vi "循环脉冲脚本.vi"(4 "4-wire":bool, 6 "脉冲":T1 {"测试参数"."反向极限电流(mA)" min=0.0 max=3000.0; "测试参数"."反向电压(V)" min=-40.0 max=40.0; "测试参数"."读取电压(V)" min=-40.0 max=40.0; "测试参数"."正向极限电流(mA)" min=0.0 max=3000.0; "测试参数"."正向电压(V)" min=-40.0 max=40.0}, 8 "错误输入（无错误）":errorcluster, 11 "循环次数":u32) -> (0 "错误输出":errorcluster, 1 "Script":string)   [LabVIEW 2020, in "功能选择.xctl"]
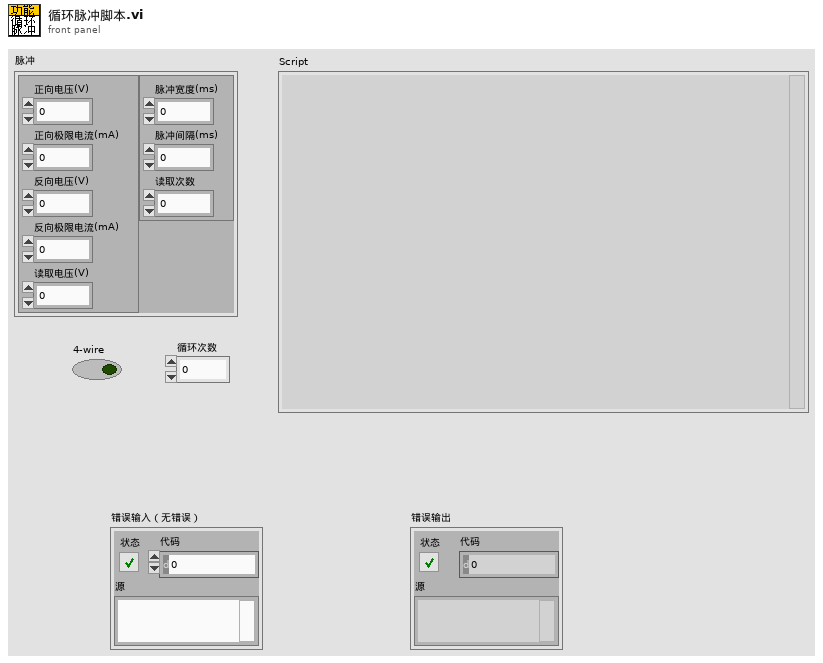
[diagram p1: front panel]
types:
  T1 = typedef "功能选择.xctl/脉冲参数.ctl" = cluster{"测试参数":cluster{"正向电压(V)":dbl, "正向极限电流(mA)":dbl, "反向电压(V)":dbl, "反向极限电流(mA)":dbl, "读取电压(V)":dbl}, "时序参数":cluster{"脉冲宽度(ms)":dbl, "脉冲间隔(ms)":dbl, "读取次数":u32}}
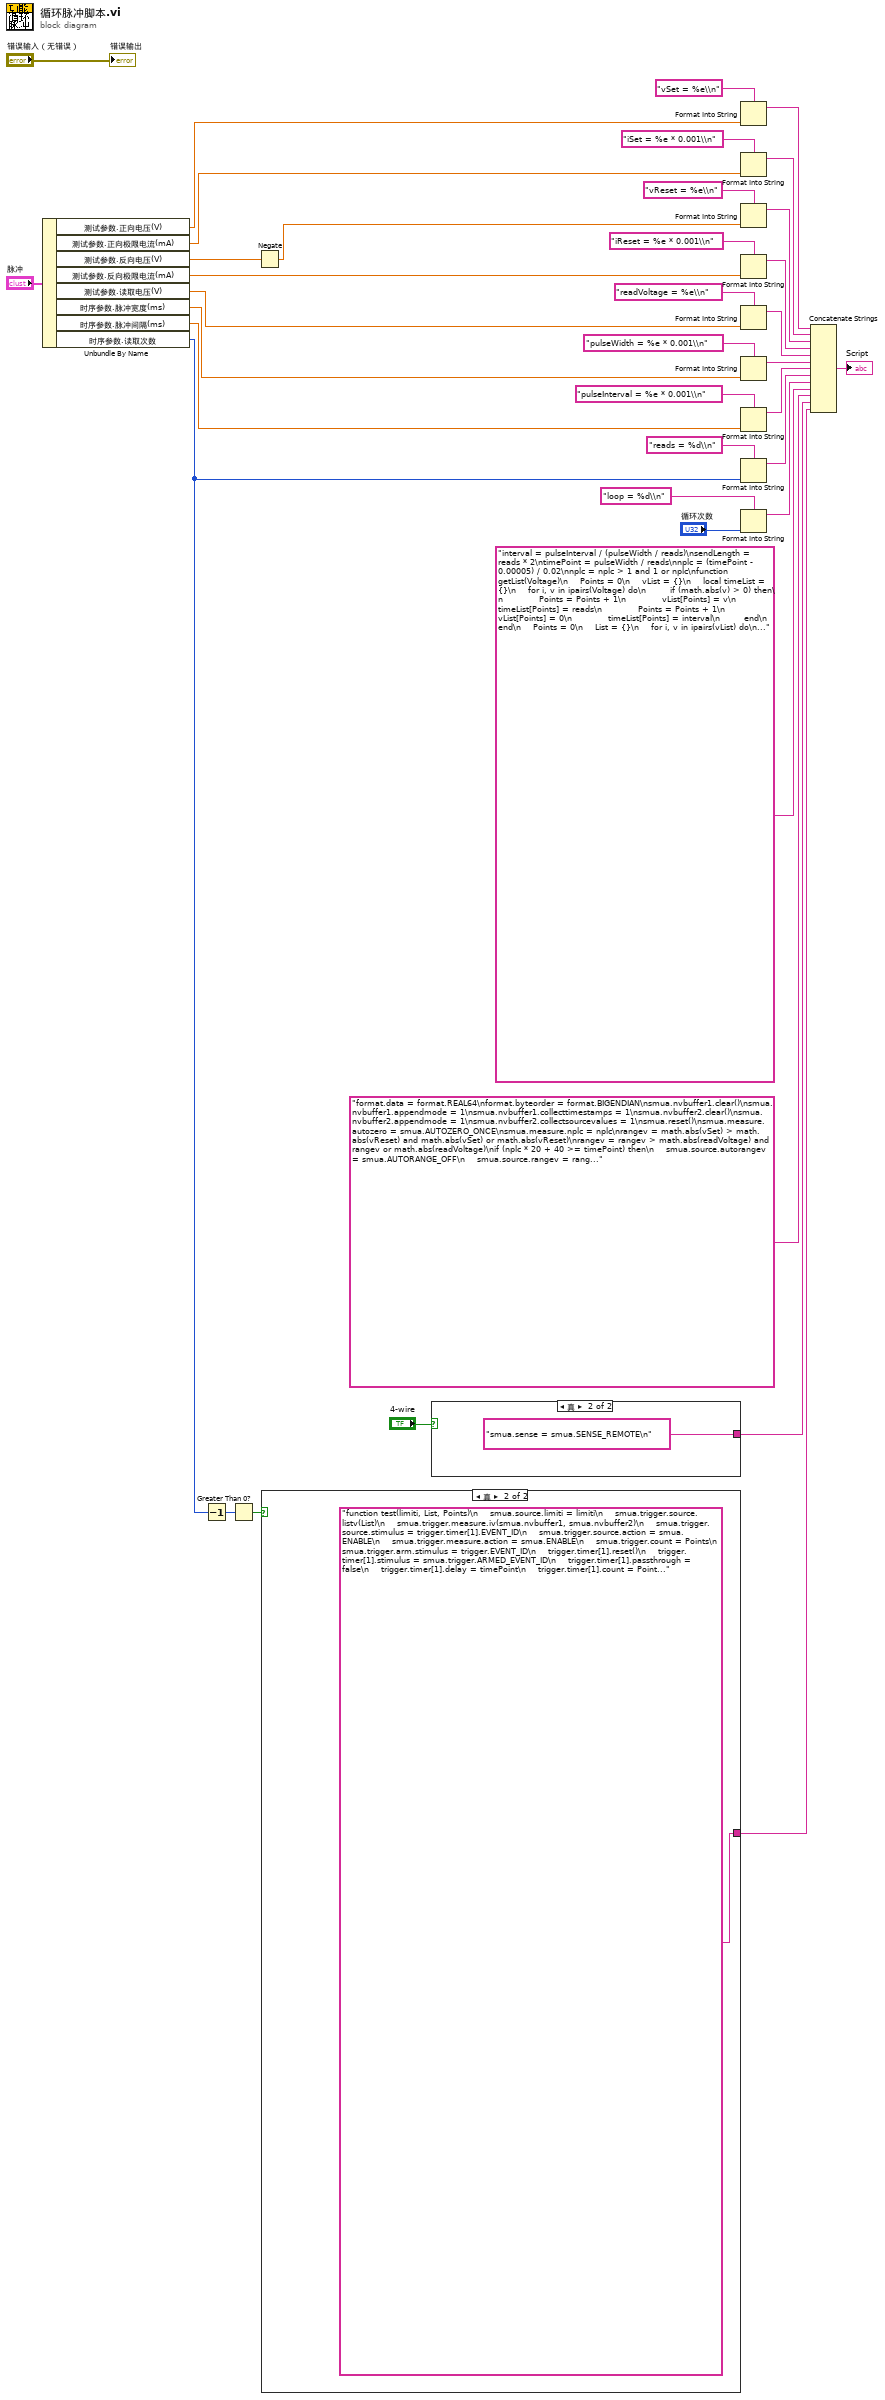
[diagram p0: block diagram]
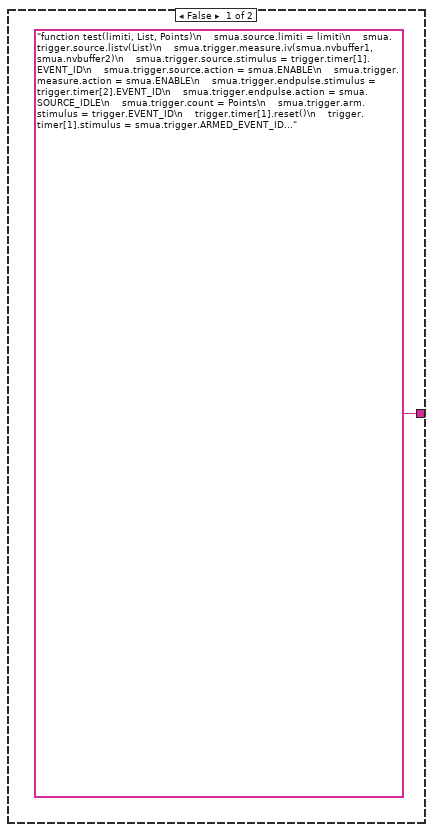
[diagram p2: hidden frame]
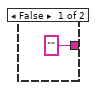
[diagram p3: hidden frame]
diagram:
  n1 = Unbundle By Name("脉冲") -> ("测试参数.正向电压(V)"=w24:dbl, "测试参数.正向极限电流(mA)"=w23:dbl, "测试参数.反向电压(V)"=w22:dbl, "测试参数.反向极限电流(mA)"=w21:dbl, "测试参数.读取电压(V)"=w30:dbl, "时序参数.脉冲宽度(ms)"=w29:dbl, "时序参数.脉冲间隔(ms)"=w2:dbl, "时序参数.读取次数"=w9:u32)
  n2 = Decrement(x=w9) -> (x-1=w10:u32)
  n3 = Greater Than 0?(x=w10) -> (x > 0?=w6:bool)
  n4 = Negate(x=w22) -> (-x=w8:dbl)
  n5 = case shown="真" w6 {
    tunnel: ["function test(limiti, List, Points)\n    smua.source.limiti = limiti\n    smua.trigger.source.listv(List)\n    smua.trigger.measure.iv(smua.nvbuffer1, smua.nvbuffer2)\n    smua.trigger.source.stimulus = trigger.timer[1].EVENT_ID\n    smua.trigger.source.action = smua.ENABLE\n    smua.trigger.measure.action = smua.ENABLE\n    smua.trigger.endpulse.stimulus = trigger.timer[2].EVENT_ID\n    smua.trigger.endpulse.action = smua.SOURCE_IDLE\n    smua.trigger.count = Points\n    smua.trigger.arm.stimulus = trigger.EVENT_ID\n    trigger.timer[1].reset()\n    trigger.timer[1].stimulus = smua.trigger.ARMED_EVENT_ID\n    trigger.timer[1].passthrough = false\n    trigger.timer[1].delay = timePoint\n    trigger.timer[1].count = Points\n    trigger.timer[2].reset()\n    trigger.timer[2].stimulus = trigger.timer[1].EVENT_ID\n    trigger.timer[2].passthrough = false\n    trigger.timer[2].delay = pulseWidth\n    trigger.timer[2].count = 1\n    smua.trigger.initiate()\n    smua.trigger.arm.set()\nend\nsmua.source.output = smua.OUTPUT_ON\nfor i = 1, loop do\n    if (setPoints > 0) then\n        test(iSet, setList, setPoints)\n        waitcomplete()\n    end\n    if (ResetPoints > 0) then\n        test(iReset, ResetList, ResetPoints)\n        waitcomplete()\n    end\nend\nsmua.source.output = smua.OUTPUT_OFF\nStart = 1\nStop = smua.nvbuffer1.n\nprint(\"{\" .. Stop .. \"}\")\nprintbuffer(Start, Stop, smua.nvbuffer1.timestamps)\nprintbuffer(Start, Stop, smua.nvbuffer2.sourcevalues)\nprintbuffer(Start, Stop, smua.nvbuffer1)\nprintbuffer(Start, Stop, smua.nvbuffer2)\nprint(\"{done}\")\nreset()" ("字符串") "function test(limiti, List, Points)\n    smua.source.limiti = limiti\n    smua.trigger.source.listv(List)\n    smua.trigger.measure.iv(smua.nvbuffer1, smua.nvbuffer2)\n    smua.trigger.source.stimulus = trigger.timer[1].EVENT_ID\n    smua.trigger.source.action = smua.ENABLE\n    smua.trigger.measure.action = smua.ENABLE\n    smua.trigger.count = Points\n    smua.trigger.arm.stimulus = trigger.EVENT_ID\n    trigger.timer[1].reset()\n    trigger.timer[1].stimulus = smua.trigger.ARMED_EVENT_ID\n    trigger.timer[1].passthrough = false\n    trigger.timer[1].delay = timePoint\n    trigger.timer[1].count = Points\n    smua.trigger.initiate()\n    smua.trigger.arm.set()\nend\nfunction sendData()\n    repeat\n        if (bit.test(status.operation.instrument.smua.condition, 4) == false) then\n            return\n        elseif (smua.nvbuffer1.n > Stop) then\n            print(\"{\" .. sendLength .. \"}\")\n            printbuffer(Start, Stop, smua.nvbuffer1.timestamps)\n            printbuffer(Start, Stop, smua.nvbuffer2.sourcevalues)\n            printbuffer(Start, Stop, smua.nvbuffer1)\n            printbuffer(Start, Stop, smua.nvbuffer2)\n            Start = Start + sendLength\n            Stop = Stop + sendLength\n        end\n        delay(timePoint)\n    until (false)\nend\nfunction sendLastData()\n    Stop = smua.nvbuffer1.n\n    print(\"{\" .. Stop - Start + 1 .. \"}\")\n    printbuffer(Start, Stop, smua.nvbuffer1.timestamps)\n    printbuffer(Start, Stop, smua.nvbuffer2.sourcevalues)\n    printbuffer(Start, Stop, smua.nvbuffer1)\n    printbuffer(Start, Stop, smua.nvbuffer2)\n    print(\"{done}\")\nend\nStart = 1\nStop = sendLength\nsmua.source.output = smua.OUTPUT_ON\ntest(iSet, startList, startPoints)\nsendData()\nfor i = 1, loop do\n    if (setPoints > 0) then\n        test(iSet, setList, setPoints)\n        sendData()\n    end\n    if (ResetPoints > 0) then\n        test(iReset, ResetList, ResetPoints)\n        sendData()\n    end\nend\nsmua.source.output = smua.OUTPUT_OFF\nsendLastData()\nreset()" ("字符串")] -> w13
    frame False {
    }
    frame True {
    }
  }
  n6 = case shown="真" "4-wire" {
    tunnel: ["" "smua.sense = smua.SENSE_REMOTE\n"] -> w36
    frame False {
    }
    frame True {
    }
  }
  n7 = Format Into String(format string="vSet = %e\\n" ("格式字符串"), w24) -> (resulting string=w20:string)  [unwired: 2 in, 1 out]
  n8 = Format Into String(format string="iSet = %e * 0.001\\n" ("格式字符串"), w23) -> (resulting string=w19:string)  [unwired: 2 in, 1 out]
  n9 = Format Into String(format string="vReset = %e\\n" ("格式字符串"), w8) -> (resulting string=w18:string)  [unwired: 2 in, 1 out]
  n10 = Format Into String(format string="iReset = %e * 0.001\\n" ("格式字符串"), w21) -> (resulting string=w17:string)  [unwired: 2 in, 1 out]
  n11 = Format Into String(format string="readVoltage = %e\\n" ("格式字符串"), w30) -> (resulting string=w16:string)  [unwired: 2 in, 1 out]
  n12 = Format Into String(format string="pulseWidth = %e * 0.001\\n", w29) -> (resulting string=w15:string)  [unwired: 2 in, 1 out]
  n13 = Format Into String(format string="pulseInterval = %e * 0.001\\n", w2) -> (resulting string=w1:string)  [unwired: 2 in, 1 out]
  n14 = Format Into String(format string="reads = %d\\n" ("格式字符串"), w9) -> (resulting string=w34:string)  [unwired: 2 in, 1 out]
  n15 = Format Into String(format string="loop = %d\\n" ("格式字符串"), "循环次数") -> (resulting string=w11:string)  [unwired: 2 in, 1 out]
  n16 = Concatenate Strings(w20, w19, w18, w17, w16, w15, w1, w34, w11, "interval = pulseInterval / (pulseWidth / reads)\nsendLength = reads * 2\ntimePoint = pulseWidth / reads\nnplc = (timePoint - 0.00005) / 0.02\nnplc = nplc > 1 and 1 or nplc\nfunction getList(Voltage)\n    Points = 0\n    vList = {}\n    local timeList = {}\n    for i, v in ipairs(Voltage) do\n        if (math.abs(v) > 0) then\n            Points = Points + 1\n            vList[Points] = v\n            timeList[Points] = reads\n            Points = Points + 1\n            vList[Points] = 0\n            timeList[Points] = interval\n        end\n    end\n    Points = 0\n    List = {}\n    for i, v in ipairs(vList) do\n        for i = 1, timeList[i] do\n            Points = Points + 1\n            List[Points] = v\n        end\n    end\n    return List, Points\nend\nstartPoints = interval\nstartList = {}\nfor i = 1, startPoints do\n    startList[i] = 0\nend\nsetList, setPoints = getList({ vSet, readVoltage })\nResetList, ResetPoints = getList({ vReset, readVoltage })\n" ("字符串"), "format.data = format.REAL64\nformat.byteorder = format.BIGENDIAN\nsmua.nvbuffer1.clear()\nsmua.nvbuffer1.appendmode = 1\nsmua.nvbuffer1.collecttimestamps = 1\nsmua.nvbuffer2.clear()\nsmua.nvbuffer2.appendmode = 1\nsmua.nvbuffer2.collectsourcevalues = 1\nsmua.reset()\nsmua.measure.autozero = smua.AUTOZERO_ONCE\nsmua.measure.nplc = nplc\nrangev = math.abs(vSet) > math.abs(vReset) and math.abs(vSet) or math.abs(vReset)\nrangev = rangev > math.abs(readVoltage) and rangev or math.abs(readVoltage)\nif (nplc * 20 + 40 >= timePoint) then\n    smua.source.autorangev = smua.AUTORANGE_OFF\n    smua.source.rangev = rangev\n    smua.measure.autorangei = smua.AUTORANGE_OFF\n    smua.measure.rangei = iSet > iReset and iSet or iReset\nend\n" ("字符串"), w36, w13) -> (→"Script":string)
  "错误输出" <- "错误输入（无错误）"
